vi "Get Global MetaData Parent Refnum.vi"(8 "error in (no error)":errorcluster, 11 "instrument addon refnum in":T1 format="%.0x") -> (0 "error out":errorcluster, 2 "global metadata section refnum":T1 format="%.0x", 3 "instrument addon refnum out":T1 format="%.0x")   [LabVIEW 2020, in "Instrument Addon Scripting API.lvlib"]
uses:
  Instrument Addon Scripting API.lvlib
  <vilib>/NI VeriStand/Custom Device API/Custom Device Item Ref.ctl
  Shared Directory/Constants.vi
  <vilib>/NI VeriStand/Custom Device Tools/Custom Device Utility Library/NI VeriStand - Search for Item by GUID.vi
  <vilib>/NI VeriStand/Custom Device Tools/Custom Device Utility Library/Custom Device Utility Library.lvlib
  Shared Directory/Instrument Addon Shared.lvlib
  <vilib>/NI VeriStand/Custom Device API/Custom Device API.lvlib
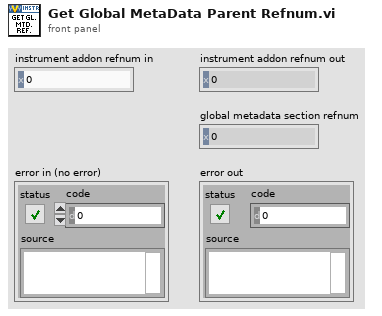
[diagram p1: front panel]
types:
  T1 = typedef "Custom Device API.lvlib/Custom Device Item Ref.ctl" = u64
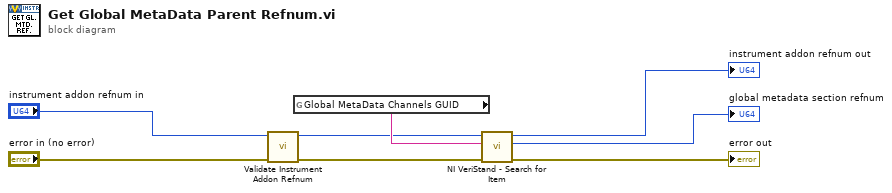
[diagram p0: block diagram]
diagram:
  n1 = call "Validate Instrument Addon Refnum.vi"("Error In"="error in (no error)", "Refnum In"="instrument addon refnum in") -> ("Error Out"=w2:errorcluster, "Refnum Out"=w1:T1)  [unwired: 7 in, 1 out]
  n2 = global read "Constants.vi" "Global MetaData Channels GUID"() -> (w3:string)
  n3 = call-poly <vilib>:"NI VeriStand - Search for Item.vi"("error in"=w2, "Item GUID"=w3, "Section Ref in"=w1) -> ("error out"=→"error out":errorcluster, "Item Ref"=→"global metadata section refnum":T1, "Section Ref out"=→"instrument addon refnum out":T1)  [unwired: 5 in, 1 out]
